vi "Test SMO Debug.vi"() -> ()   [LabVIEW 2019]
uses:
  subsystems/Attribute.Debug/DebugBehavior.ctl
  <vilib>/JKI/JKI SMO/SMO/SMO.lvclass
  Debug.lvlib
  subsystems/Attribute.Debug/Attribute.Debug.lvclass
panel:
  in  "Behavior":T1
  out "Behavior":T1
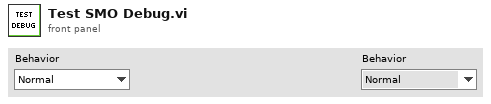
[diagram p1: front panel]
types:
  T1 = typedef "Debug.lvlib/Attribute.Debug.lvclass/DebugBehavior.ctl" = enum16{"Normal", "Debug"}
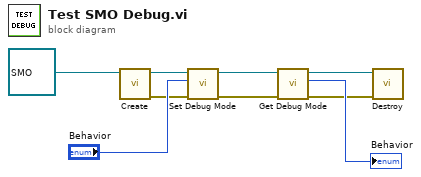
[diagram p0: block diagram]
diagram:
  n1 = call <vilib>:"Create.vi"("SMO"=refnum<class "SMO.lvclass"> refnum) -> ("error out"=w4:errorcluster, "SMO out"=w6:refnum<class "SMO.lvclass">)  [unwired: 8 in, 1 out]
  n2 = call "Set Debug Mode.vi"("error in (no error)"=w4, "Behavior"="Behavior", "SMO"=w6) -> ("error out"=w3:errorcluster, "SMO out"=w1:refnum<class "SMO.lvclass">)  [unwired: 7 in]
  n3 = call "Get Debug Mode.vi"("error in (no error)"=w3, "SMO"=w1) -> ("error out"=w2:errorcluster, "Behavior"=→"Behavior":T1, "SMO out"=w8:refnum<class "SMO.lvclass">)  [unwired: 7 in]
  n4 = call <vilib>:"Destroy.vi"("error in (no error)"=w2, "SMO"=w8) -> ()  [unwired: 9 in, 1 out]
